vi "LBCB Read.vi"(4 "error in (no error)":errorcluster, 6 "Container State":T6, 7 "Display State In":T1) -> (0 "error out":errorcluster, 2 "Value":T4, 3 "Display State Out":T1)   [LabVIEW 2013, in "Limits X.xctl"]
uses:
  Limits X.xctl
  <vilib>/_xctls/Container State.ctl
  lib/Data Access Objects/Metadata/LBCB Number.ctl
  Limits State.ctl
  lib/Data Access Objects/Limits/DofTypes.ctl
  lib/Limits/Limite State.ctl
  lib/Apps/Yes No Button.ctl
  <vilib>/_xctls/XControlSupport.lvlib
panel:
  # "Replace the Value Indicator below with an Indicator of desired type.\nDo not remove this Indicator or the others from the connector pane. \nDo not change the connector pane pattern.\nThe Value Indicator should always be the second terminal from top on the output side in the connector pane."
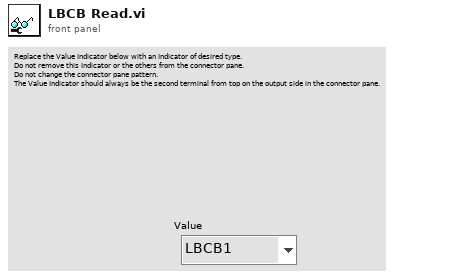
[diagram p1: front panel]
types:
  T1 = typedef "Limits X.xctl/Limits State.ctl" = cluster{"DofType":T2, "Limit State":T3, "LBCB Number":T4, "DOF Index":i32, "System Fault ":T5, "Has Lower":T5}
  T2 = typedef "DofTypes.ctl" = enum16{"Cartesian Displacements", "Cartesian Forces & Moments", "Actuator Displacements", "Actuator Forces", "Cartesian Increments", "Actuator Increments"}
  T3 = typedef "Limite State.ctl" = enum16{"Good", "Lower Bound Fault", "Upper Bound Fault"}
  T4 = typedef "LBCB Number.ctl" = enum16{"LBCB1", "LBCB2"}
  T5 = typedef "Yes No Button.ctl" = bool
  T6 = typedef "XControlSupport.lvlib/Container State.ctl" = cluster{"Indicator?":bool, "Run Mode?":bool, " Refnum":refnum<vi>}
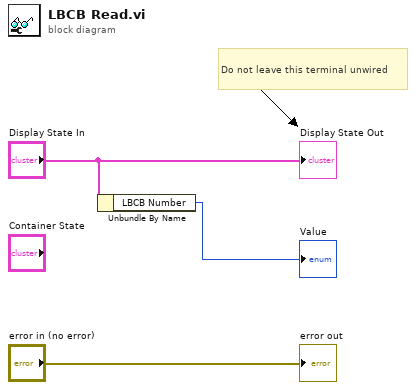
[diagram p0: block diagram]
diagram:
  # "Do not leave this terminal unwired"
  n1 = Unbundle By Name("Display State In") -> ("LBCB Number"=→"Value":T4)
  "error out" <- "error in (no error)"
  "Display State Out" <- "Display State In"
